vi "finalize initialization.vi"(8 "error in":errorcluster, 10 "configuration in":refnum<class "fixed channel configuration.lvclass">, 11 "fixed channel tag bus module in":refnum<class "fixed channel tag bus module.lvclass">) -> (0 "error out":errorcluster, 3 "fixed channel tag bus module out":refnum<class "fixed channel tag bus module.lvclass">)   [LabVIEW 2013, in "fixed channel tag bus module.lvclass"]
uses:
  fixed channel tag bus module.lvclass
  fixed module parent/module/configuration/fixed channel configuration.lvclass
  configuration/fixed channel tag bus module configuration.lvclass
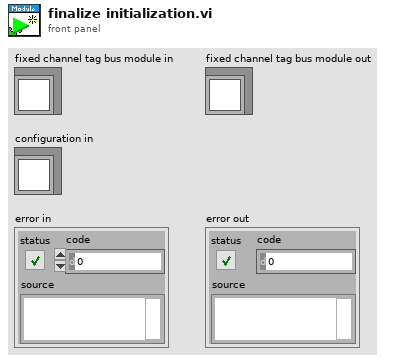
[diagram p1: front panel]
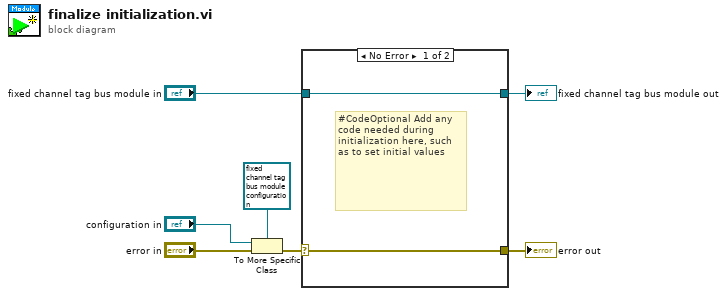
[diagram p0: block diagram]
diagram:
  n1 = To More Specific Class(target class=refnum<class "fixed channel tag bus module configuration.lvclass"> refnum ("user module configuration"), reference="configuration in", error in="error in") -> (error out=w4:errorcluster)  [unwired: 1 out]
  n2 = case shown="No Error" w4 {
    selector: w4 -> [w8 w10]
    tunnel: [w9 w11] -> w3
    tunnel: "fixed channel tag bus module in" -> [w9 w11]
    tunnel: [w8 w10] -> w1
    frame No Error {
      # "#CodeOptional Add any code needed during initialization here, such as to set initial values"
    }
    frame Error {
    }
  }
  "error out" <- w1
  "fixed channel tag bus module out" <- w3
